vi "mvgpdf.vi"(8 "input_ERP(normalized)":dbl[](array[numeric]), 11 "covariance":dbl[][](array[numeric])) -> (3 "Gaussian_prob":ext)   [LabVIEW 2013]
uses:
  <vilib>/Analysis/baseanly.llb/Real A x B.vi
  <vilib>/Analysis/baseanly.llb/Real Inverse Matrix.vi
  <vilib>/Analysis/Matrix/Numeric/Conversions/Array To Matrix - RA.vi
  <vilib>/Analysis/Matrix/Numeric/Exponential/Exponential - RM.vi
  <vilib>/Analysis/NI_AALBase.lvlib
  <vilib>/Analysis/Matrix/NI_Matrix.lvlib
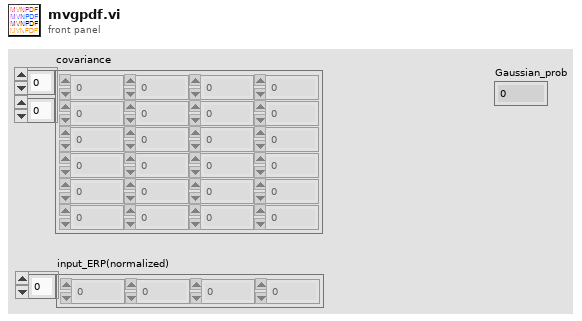
[diagram p1: front panel]
types:
  T1 = typedef "NI_Matrix.lvlib/RealMatrix.ctl" = dbl[][]
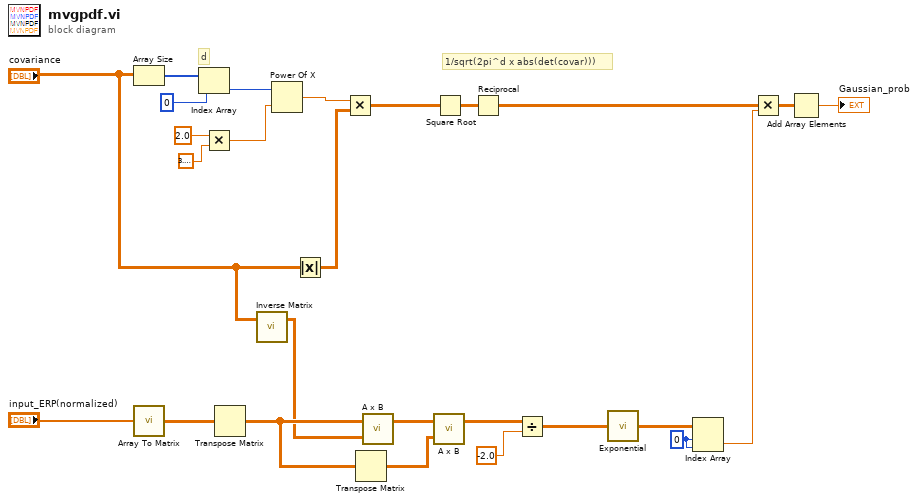
[diagram p0: block diagram]
diagram:
  w9 = 0 ("index (row)")
  # "1/sqrt(2pi^d x abs(det(covar)))"
  # "d"
  n1 = Array Size(array="covariance") -> (size(s)=w26:i32[])
  n2 = call-poly <vilib>:"Array To Matrix.vi"("Real 1D Array"="input_ERP(normalized)") -> ("Real Matrix (Column Vector)"=w12:T1)
  n3 = Index Array(array=w26, index=0) -> (element=w21:i32)
  n4 = Multiply(x=2.0, y=3.141592653589793) -> (x*y=w22:dbl)
  n5 = Transpose Matrix(1:w12) -> (0:w11:T1)
  n6 = call-poly <vilib>:"Inverse Matrix.vi"("Input Matrix"="covariance") -> ("Inverse Matrix"=w7:T1)  [unwired: 1 in, 1 out]
  n7 = Power Of X(1:w22, 2:w21) -> (0:w20:dbl)
  n8 = Absolute Value ("Absolute Value.vi")(x="covariance") -> (abs(x)=w19:dbl[][])
  n9 = Multiply ("Multiply.vi")(x=w20, y=w19) -> (x*y=w1:dbl[][])
  n10 = Transpose Matrix(1:w11) -> (0:w15:T1)
  n11 = call-poly <vilib>:"A x B.vi"("B"=w7, "A"=w11) -> ("A x B"=w16:T1)  [unwired: 1 out]
  n12 = call-poly <vilib>:"A x B.vi"("B"=w15, "A"=w16) -> ("A x B"=w6:T1)  [unwired: 1 out]
  n13 = Square Root ("Square Root.vi")(x=w1) -> (sqrt(x)=w18:dbl[][])
  n14 = Reciprocal(x=w18) -> (1/x=w4:dbl[][])
  n15 = Divide(x=w6, y=-2.0) -> (x/y=w13:T1)
  n16 = call-poly <vilib>:"Exponential.vi"("Real Matrix A"=w13) -> ("e^A"=w10:T1)
  n17 = Index Array(array=w10, index (row)=w9, index (col)=w9) -> (element=w8:dbl)
  n18 = Multiply ("Multiply.vi")(x=w4, y=w8) -> (x*y=w5:dbl[][])
  n19 = Add Array Elements(numeric array=w5) -> (sum=→"Gaussian_prob":dbl)
